vi "Actor Core.vi"(8 "error in":errorcluster, 11 "OneButtonDialogBox In":refnum<class "KeypadDialogBox.lvclass">) -> (0 "error out":errorcluster, 3 "Actor out":refnum<class "Actor.lvclass">)   [LabVIEW 2015, in "KeypadDialogBox.lvlib" / "KeypadDialogBox.lvclass"]
doc: "(<B>Filename</B>: Actor Framework.lvlib:Actor.lvclass:Actor Core.vi)\n\nReceives messages to the actor, reacts to them, and initiates any error handling that may shut the actor down.\n\nDescendant classes may override this VI to append parallel tasks for the actor to complete while it handles messages. Overrides use the Call Parent Method node."
uses:
  KeypadDialogBox.lvclass
  <vilib>/ActorFramework/Actor/Actor.lvclass
  <vilib>/event_ctls.llb/lveventtype.ctl
  KeypadDialogBox.lvclass/KeypadDialogBox.ctl
  Framework/IDialogBox/IDialogBox/IDialogBox.lvclass
  Framework/ActorEvents/IEventAggregator/IEventAggregator.lvclass
panel:
  out "Message Text":string
  in  "Value":string
  in  "Cancel":bool
  in  "OK":bool
  in  "Backspace":bool
  in  ".":bool
  in  "0":bool
  in  "9":bool
  in  "8":bool
  in  "7":bool
  in  "6":bool
  in  "5":bool
  in  "4":bool
  in  "3":bool
  in  "2":bool
  in  "1":bool
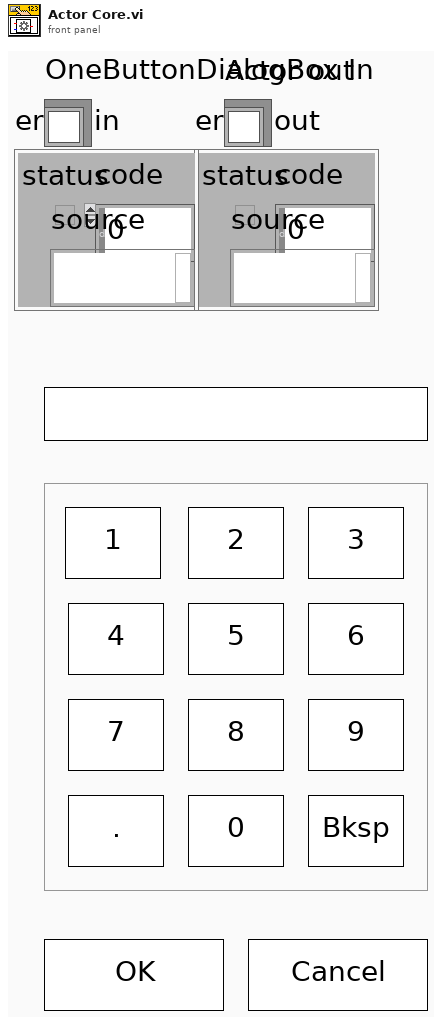
[diagram p1: front panel]
types:
  T1 = typedef "lveventtype.ctl" = enum32{"Null", "Timeout", "Annotation Menu Selection", "Annotation Menu Selection?", "App Instance Close", "App Instance Close?", "Autoscale Range Change", "Bookmark Info Change", "Cell Edit", "Cell Edit?", "Cursor Grab", "Cursor Grab?", "Cursor Menu Selection", "Cursor Menu Selection?", "Cursor Move", "Cursor Release", "Data Change", "Direction Change", "Display State Change", "Drag Ended", "Drag Enter", "Drag Leave", "Drag Over", "Drag Source Update", "Drag Starting", "Drag Starting?", "Drop", "Exec State Change", "Key Down", "Key Down?", "Key Repeat", "Key Repeat?", "Key Up", "Listbox Double Click", "Menu Activation?", "Menu Selection (App)", "Menu Selection? (App)", "Menu Selection (User)", "Mouse Down", "Mouse Down?", "Mouse Enter", "Mouse Leave", "Mouse Move", "Mouse Up", "Mouse Wheel", "NI Security User Change (App)", "Pane Size", "Panel Close", "Panel Close?", "Panel Resize", "Plot Attribute Change", "Scale Range Change", "Shortcut Menu Activation?", "Shortcut Menu Selection (App)", "Shortcut Menu Selection? (App)", "Shortcut Menu Selection (User)", "Tree Double Click", "Tree Drag", "Tree Drag?", "Tree Drop", "Tree Drop?", "Tree Item Close", "Tree Item Close?", "Tree Item Open", "Tree Item Open?", "User Event", "Value Change"}
  T2 = enum32{"Invalid", "Default", "Floating", "Floating/Auto-Hide", "Modal"}
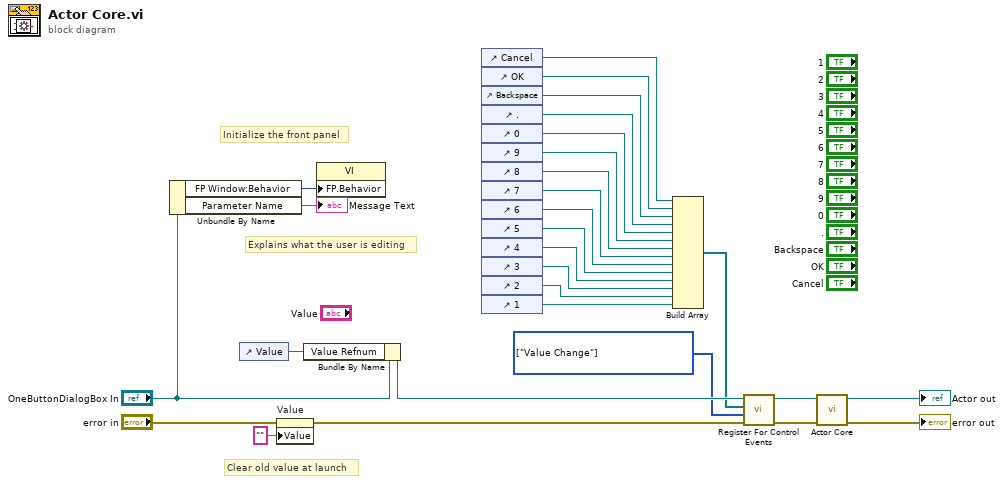
[diagram p0: block diagram]
diagram:
  w1 = T1[] [enum."Value Change"] items=["Null", "Timeout", "Annotation Menu Selection", "Annotation Menu Selection?", "App Instance Close", "App Instance Close?", "Autoscale Range Change", "Bookmark Info Change", "Cell Edit", "Cell Edit?", "Cursor Grab", "Cursor Grab?", "Cursor Menu Selection", "Cursor Menu Selection?", "Cursor Move", "Cursor Release", "Data Change", "Direction Change", "Display State Change", "Drag Ended", "Drag Enter", "Drag Leave", "Drag Over", "Drag Source Update", "Drag Starting", "Drag Starting?", "Drop", "Exec State Change", "Key Down", "Key Down?", "Key Repeat", "Key Repeat?", "Key Up", "Listbox Double Click", "Menu Activation?", "Menu Selection (App)", "Menu Selection? (App)", "Menu Selection (User)", "Mouse Down", "Mouse Down?", "Mouse Enter", "Mouse Leave", "Mouse Move", "Mouse Up", "Mouse Wheel", "NI Security User Change (App)", "Pane Size", "Panel Close", "Panel Close?", "Panel Resize", "Plot Attribute Change", "Scale Range Change", "Shortcut Menu Activation?", "Shortcut Menu Selection (App)", "Shortcut Menu Selection? (App)", "Shortcut Menu Selection (User)", "Tree Double Click", "Tree Drag", "Tree Drag?", "Tree Drop", "Tree Drop?", "Tree Item Close", "Tree Item Close?", "Tree Item Open", "Tree Item Open?", "User Event", "Value Change"] ("Registration Types")
  # "Explains what the user is editing"
  # "Clear old value at launch"
  # "Initialize the front panel"
  n1 = Unbundle By Name("OneButtonDialogBox In") -> ("FP Window:Behavior"=w27:T2, "Parameter Name"=→"Message Text":string)
  n2 = control-ref of="Value"() -> (w23:refnum<vi>)
  n3 = property on="Value" class="Str"(error in="error in", "Value"="") -> (error out=w18:errorcluster)  [unwired: 1 in, 1 out]
  n4 = Bundle By Name(cluster="OneButtonDialogBox In", "Value Refnum"=w23) -> (w24:refnum<class "KeypadDialogBox.lvclass">)
  n5 = property class="VI"("FP.Behavior"=w27) -> ()  [unwired: 2 in, 2 out]
  n6 = control-ref of="Cancel"() -> (w16:refnum<vi>)
  n7 = control-ref of="OK"() -> (w15:refnum<vi>)
  n8 = control-ref of="Backspace"() -> (w14:refnum<vi>)
  n9 = control-ref of="."() -> (w13:refnum<vi>)
  n10 = control-ref of="0"() -> (w12:refnum<vi>)
  n11 = control-ref of="9"() -> (w11:refnum<vi>)
  n12 = control-ref of="8"() -> (w10:refnum<vi>)
  n13 = control-ref of="7"() -> (w9:refnum<vi>)
  n14 = control-ref of="6"() -> (w8:refnum<vi>)
  n15 = control-ref of="5"() -> (w7:refnum<vi>)
  n16 = control-ref of="4"() -> (w6:refnum<vi>)
  n17 = control-ref of="3"() -> (w5:refnum<vi>)
  n18 = control-ref of="2"() -> (w4:refnum<vi>)
  n19 = control-ref of="1"() -> (w3:refnum<vi>)
  n20 = Build Array(w16, w15, w14, w13, w12, w11, w10, w9, w8, w7, w6, w5, w4, w3) -> (w2:refnum<vi>[])
  n21 = call "Register For Control Events.vi"("error in (no error)"=w18, "Registration Types"=w1, "Control Refnums"=w2, "IEventAggregator In"=w24) -> ("error out"=w17:errorcluster, "IEventAggregator Out"=w19:refnum<class "KeypadDialogBox.lvclass">)  [unwired: 6 in]
  n22 = call-parent "Actor Core.vi"("error in"=w17, "IViewable In"=w19) -> ("error out"=→"error out":errorcluster, "Actor out"=→"Actor out":refnum<class "Actor.lvclass">)  [unwired: 8 in]
